vi "log.vi"(8 "error in (no error)":errorcluster, 10 "Message":string, 11 "Mission in":refnum<class "GenericMission.lvclass">) -> (0 "error out":errorcluster, 3 "Mission out":refnum<class "GenericMission.lvclass">)   [LabVIEW 2011, in "GenericMission.lvclass"]
doc: "Writes a log string to internal storage of the mission with an attached timestamp."
uses:
  GenericMission.lvclass
  2 Globals/2 Message Logger.vi
  Logger/Logger.lvclass
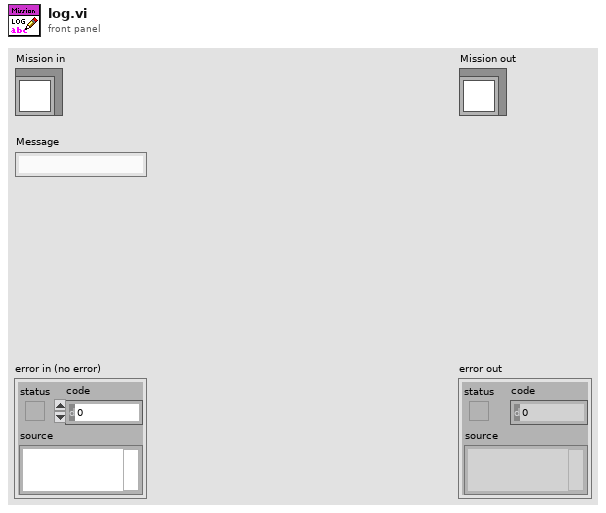
[diagram p1: front panel]
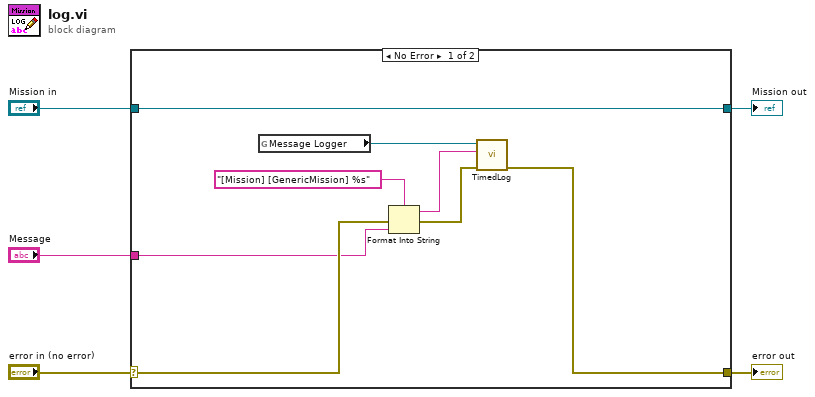
[diagram p0: block diagram]
diagram:
  n1 = case shown="No Error" "error in (no error)" {
    selector: "error in (no error)" -> [w13 w15]
    tunnel: [w8 w15] -> w4
    tunnel: [w12 w14] -> w2
    tunnel: "Mission in" -> [w12 w14]
    tunnel: "Message" -> [w6 _]
    frame No Error {
      n2 = global read "2 Message Logger.vi" "Message Logger"() -> (w11:refnum<class "Logger.lvclass">)
      n3 = Format Into String(format string="[Mission] [GenericMission] %s", error in=w13, w6) -> (resulting string=w10:string, error out=w9:errorcluster)  [unwired: 1 in]
      n4 = call "TimedLog.vi"("error in (no error)"=w9, "Message"=w10, "Logger in"=w11) -> ("error out"=w8:errorcluster)  [unwired: 6 in, 2 out]
    }
    frame Error {
    }
  }
  "error out" <- w4
  "Mission out" <- w2
